vi "Ejercicio 2.3 Tanque y temperatura.vi"() -> ()   [LabVIEW 2020]
panel:
  in  "stop":bool
  out "ALERTA PEGRILOSO":bool
  out "Termòmetro":dbl(slide) scale=0.0..100.0
  out "Tanque de agua":dbl(slide) scale=0.0..10.0
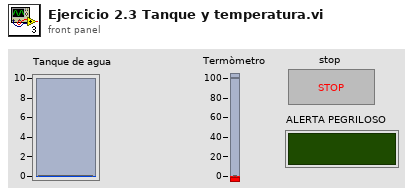
[diagram p1: front panel]
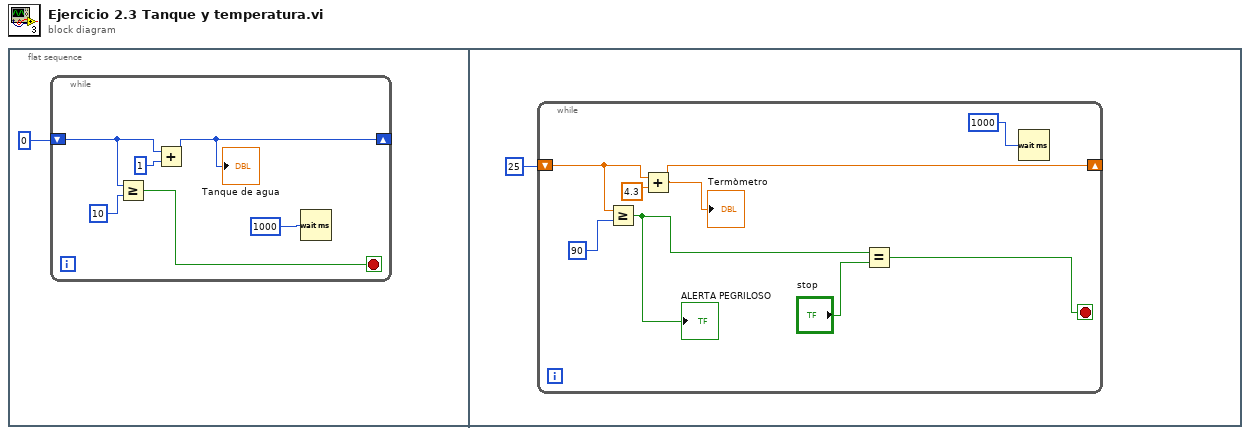
[diagram p0: block diagram]
diagram:
  n1 = flat-sequence {
    frame #0 {
      n2 = while {
        shift-right: [w4] -> _
        shift-left: 0 -> [w3]
        stop <- w7 stop-if-true
        n3 = Greater Or Equal?(x=w3, y=10) -> (x >= y?=w7:bool)
        n4 = Add(x=w3, y=1) -> (x+y=w4:i32)
        "Tanque de agua" <- w4
        n5 = Wait (ms)(milliseconds to wait=u32 1000) -> ()  [unwired: 1 out]
      }
    }
    frame #1 {
      n6 = while {
        shift-right: [w13] -> _
        shift-left: 25 -> [w15]
        stop <- w9 stop-if-true
        n7 = Greater Or Equal?(x=w15, y=90) -> (x >= y?=w11:bool)
        "ALERTA PEGRILOSO" <- w11
        n8 = Add(x=w15, y=4.3) -> (x+y=w13:dbl)
        "Termòmetro" <- w13
        n9 = Equal?(x=w11, y="stop") -> (x = y?=w9:bool)
        n10 = Wait (ms)(milliseconds to wait=u32 1000) -> ()  [unwired: 1 out]
      }
    }
  }
